vi "Set Properties.vi"(5 "Property Values":variant[](array[variant]), 7 "Property Names":string[](array[string]), 8 "error in (no error)":errorcluster, 9 "Channel Name":string, 10 "Group Name":string, 11 "Data Logger Interface in":refnum<class "TDMS Data Logger Actor.lvclass">) -> (0 "error out":errorcluster, 3 "Data Logger Interface out":refnum<class "TDMS Data Logger Actor.lvclass">)   [LabVIEW 2024, in "TDMS Data Logger Actor.lvlib" / "TDMS Data Logger Actor.lvclass"]
uses:
  TDMS Data Logger Actor.lvclass
  TDMS Data Logger Actor.lvclass/TDMS Data Logger Actor.ctl
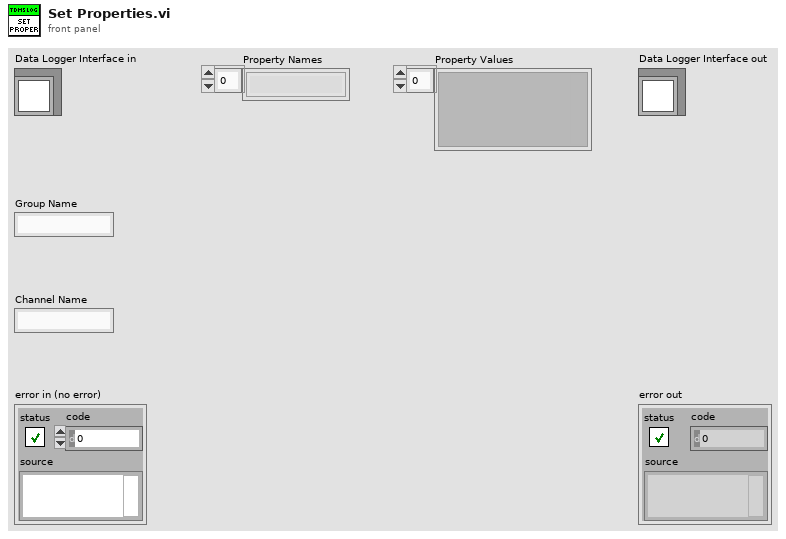
[diagram p1: front panel]
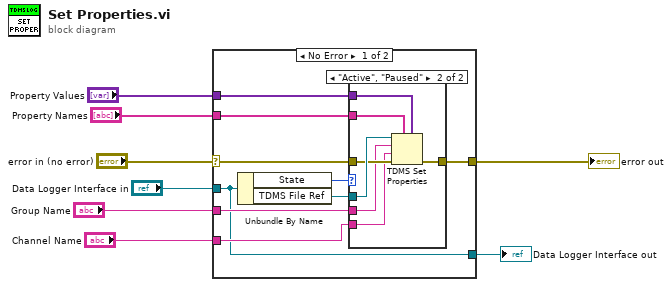
[diagram p0: block diagram]
diagram:
  n1 = case shown="No Error" "error in (no error)" {
    selector: "error in (no error)" -> [w15 w27]
    tunnel: "Data Logger Interface in" -> [w9 w26]
    tunnel: "Property Names" -> [w14 _]
    tunnel: "Property Values" -> [w13 _]
    tunnel: "Channel Name" -> [w12 _]
    tunnel: "Group Name" -> [w11 _]
    tunnel: [w10 w27] -> w2
    tunnel: [w9 w26] -> w1
    frame No Error {
      n2 = Unbundle By Name(w9) -> ("State"=w17:enum16{"Idle", "Active", "Paused"}, "TDMS File Ref"=w16:refnum<k34>)
      n3 = case shown="\"Active\", \"Paused\"" w17 {
        tunnel: w16 -> [_ w25]
        tunnel: w15 -> [w18 w24]
        tunnel: w14 -> [_ w23]
        tunnel: w13 -> [_ w22]
        tunnel: w12 -> [_ w21]
        tunnel: w11 -> [_ w20]
        tunnel: [w18 w19] -> w10
        frame "Idle" {
        }
        frame "Active", "Paused" {
          n4 = TDMS Set Properties(5:w22, 7:w23, 8:w24, 9:w21, 10:w20, 11:w25) -> (0:w19:errorcluster)  [unwired: 3 out]
        }
      }
    }
    frame Error {
    }
  }
  "error out" <- w2
  "Data Logger Interface out" <- w1
